vi "getName.vi"(8 "error in (no error)":errorcluster, 11 "IArgumentInfo in":refnum<class "IArgumentInfo.lvclass">) -> (0 "error out":errorcluster, 2 "Name out":string, 3 "IArgumentInfo out":refnum<class "IArgumentInfo.lvclass">)   [LabVIEW 2022 SP3, in "openDAQ.lvlib" / "IBaseObject.lvlib" / "IArgumentInfo.lvlib" / "IArgumentInfo.lvclass"]
uses:
  <instrlib>/openDAQ/Public/Classes/IArgumentInfo/IArgumentInfo.lvclass
  <instrlib>/openDAQ/Public/Classes/IArgumentInfo/IArgumentInfo.lvclass/IArgumentInfo.ctl
  <instrlib>/openDAQ/Public/Classes/daqCoreTypes/IString/IString.lvclass
  <instrlib>/openDAQ/Binaries/Windows/x86/copendaq32.dll
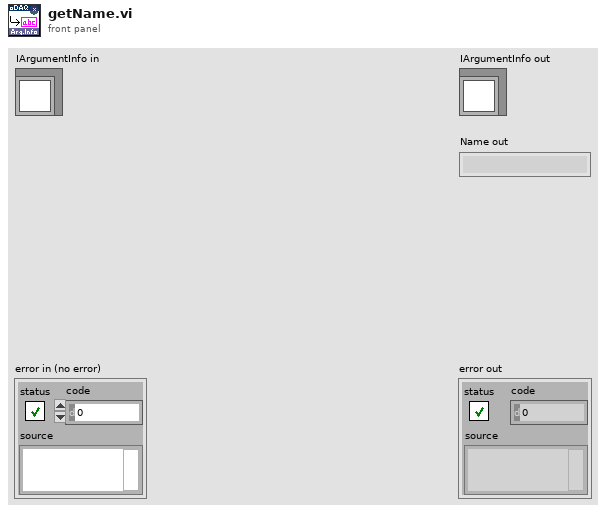
[diagram p1: front panel]
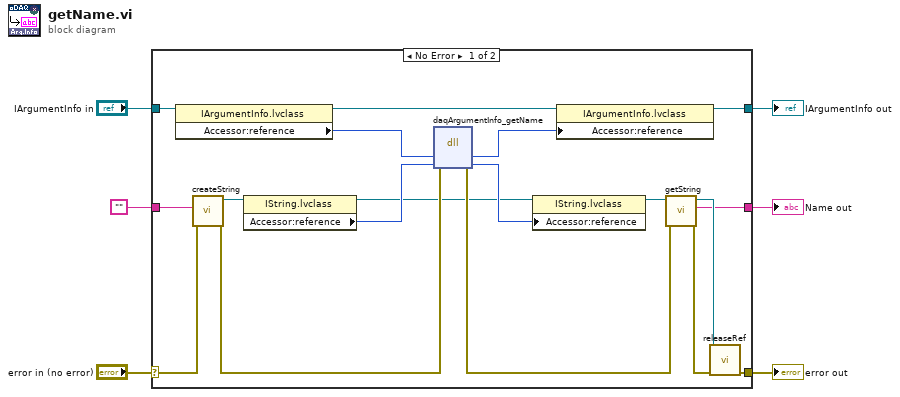
[diagram p0: block diagram]
diagram:
  n1 = case shown="No Error" "error in (no error)" {
    selector: "error in (no error)" -> [w8 w27]
    tunnel: [w11 w27] -> w5
    tunnel: [w18 w26] -> w3
    tunnel: "IArgumentInfo in" -> [w20 w26]
    tunnel: "" -> [w14 w25]
    tunnel: [w9 w25] -> w1
    frame No Error {
      n2 = property class="IArgumentInfo.lvclass"(reference=w20) -> (reference out=w19:refnum<class "IArgumentInfo.lvclass">, "Accessor:reference"=w13:i64)  [unwired: 1 in, 1 out]
      n3 = call <instrlib>:"createString.vi"("error in (no error)"=w8, "String"=w14) -> ("error out"=w24:errorcluster, "IString out"=w16:refnum<class "IString.lvclass">)  [unwired: 8 in]
      n4 = property class="IString.lvclass"(reference=w16) -> (reference out=w17:refnum<class "IString.lvclass">, "Accessor:reference"=w22:i64)  [unwired: 1 in, 1 out]
      n5 = dll-call lib="C:/Program Files (x86)/National Instruments/LabVIEW 2022/instr.lib/openDAQ/Binaries/Windows/x86/copendaq*.*" fn="daqArgumentInfo_getName"(error in=w24, "argument"=w13, "name"=w22) -> (error out=w23:errorcluster, "argument"=w12:i64, "name"=w21:i64)  [unwired: 3 in, 1 out]
      n6 = property class="IString.lvclass"(reference=w17, "Accessor:reference"=w21) -> (reference out=w15:refnum<class "IString.lvclass">)  [unwired: 1 in, 1 out]
      n7 = property class="IArgumentInfo.lvclass"(reference=w19, "Accessor:reference"=w12) -> (reference out=w18:refnum<class "IArgumentInfo.lvclass">)  [unwired: 1 in, 1 out]
      n8 = call <instrlib>:"getString.vi"("error in (no error)"=w23, "IString in"=w15) -> ("error out"=w7:errorcluster, "String out"=w9:string, "IString out"=w10:refnum<class "IString.lvclass">)  [unwired: 7 in]
      n9 = call-dynamic "releaseRef.vi"("error in (no error)"=w7, "IBaseObject in"=w10) -> ("error out"=w11:errorcluster)  [unwired: 9 in]
    }
    frame Error {
    }
  }
  "error out" <- w5
  "IArgumentInfo out" <- w3
  "Name out" <- w1
